vi "startup data collection.vi"(0 "Refnum in":T1, 1 "To Date":timestamp, 2 "Form Date":timestamp, 3 "Report filter":string, 5 "Shift":string, 7 "Select Line":string, 9 "columns":string[](array[string]), 11 "error in (no error)":errorcluster, 12 "Select Year":string, 13 "Select Month":string, 14 "table":string) -> (4 "Refnum out":T1, 6 "Array":string[](array[string]), 8 "Elements Found out":string[](array[string]), 10 "size(s)":i32, 15 "error out":errorcluster)   [LabVIEW 2017]
uses:
  <vilib>/addons/database/Connection.llb/Conn ObjectReference.ctl
  <vilib>/addons/database/NI_Database_API.lvlib
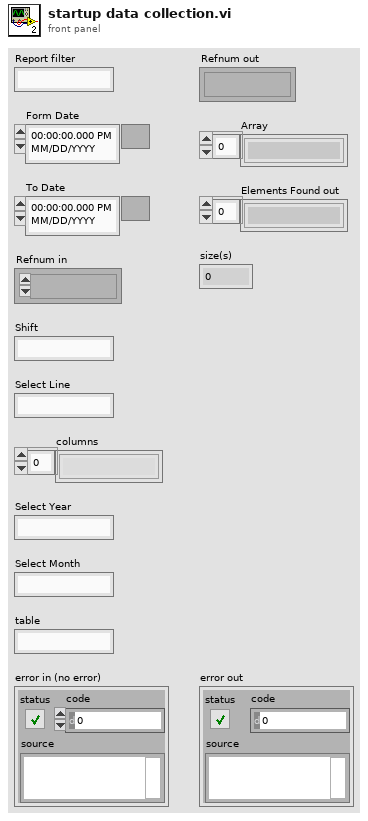
[diagram p1: front panel]
types:
  T1 = typedef "NI_Database_API.lvlib/Conn ObjectReference.ctl" = refnum<k1>
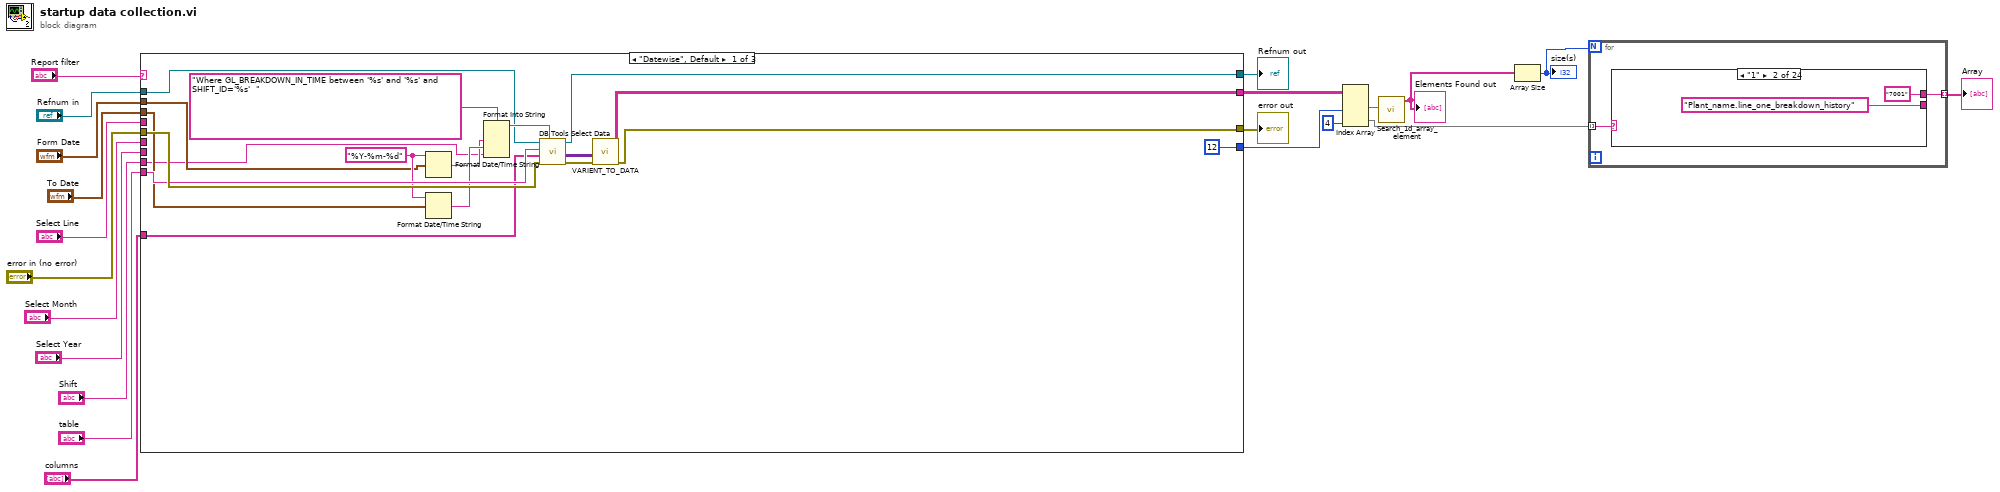
[diagram p0: block diagram]
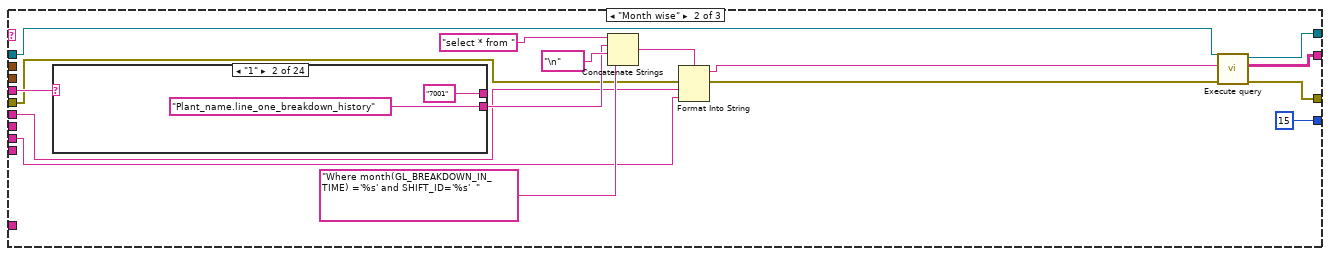
[diagram p2: hidden frame]
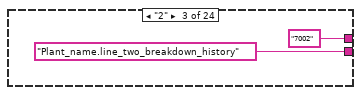
[diagram p4: hidden frame]
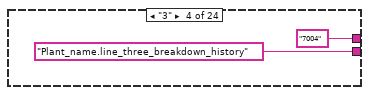
[diagram p5: hidden frame]
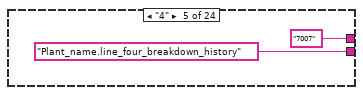
[diagram p6: hidden frame]
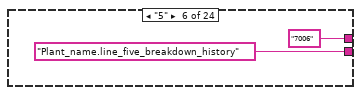
[diagram p7: hidden frame]
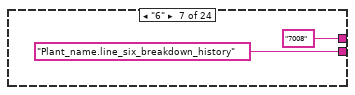
[diagram p8: hidden frame]
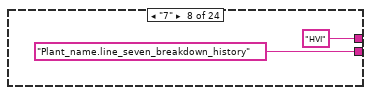
[diagram p9: hidden frame]
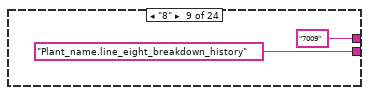
[diagram p10: hidden frame]
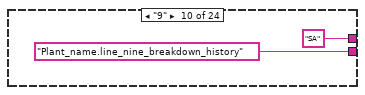
[diagram p11: hidden frame]
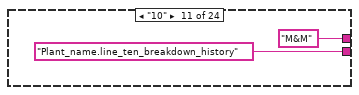
[diagram p12: hidden frame]
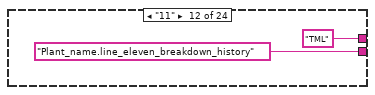
[diagram p13: hidden frame]
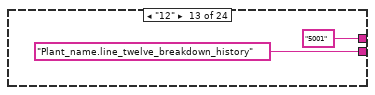
[diagram p14: hidden frame]
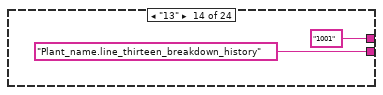
[diagram p15: hidden frame]
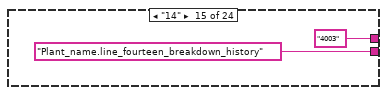
[diagram p16: hidden frame]
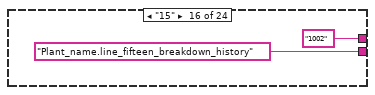
[diagram p17: hidden frame]
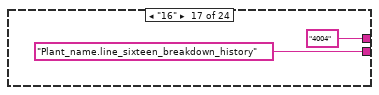
[diagram p18: hidden frame]
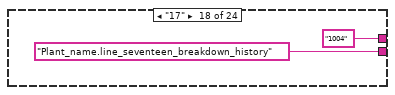
[diagram p19: hidden frame]
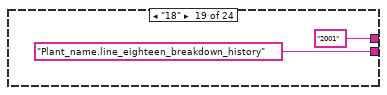
[diagram p20: hidden frame]
diagram:
  n1 = case shown="\"Datewise\", Default" "Report filter" {
    tunnel: [w37 w49 w102] -> w1
    tunnel: "Refnum in" -> [w36 w46 w113]
    tunnel: [w35 w48 w114] -> w9
    tunnel: "error in (no error)" -> [w34 w41 w109]
    tunnel: "table" -> [w33 _ _]
    tunnel: "columns" -> [w32 _ _]
    tunnel: [w30 w43 w112] -> w13
    tunnel: "Form Date" -> [w25 _ _]
    tunnel: "To Date" -> [w24 _ _]
    tunnel: "Shift" -> [w23 w45 w107]
    tunnel: "Select Line" -> [_ w51 w104]
    tunnel: "Select Month" -> [_ w44 _]
    tunnel: [12 ("disabled index (col)") 15 ("disabled index (col)") 15 ("disabled index (col)")] -> w20
    tunnel: "Select Year" -> [_ _ w108]
    frame "Datewise", Default {
      w29 = "%Y-%m-%d" ("time format string (%c)")
      n2 = Format Date/Time String(time format string (%c)=w29, seconds (now)=w25) -> (date/time string=w27:string)  [unwired: 1 in]
      n3 = Format Date/Time String(time format string (%c)=w29, seconds (now)=w24) -> (date/time string=w28:string)  [unwired: 1 in]
      n4 = Format Into String(format string="Where GL_BREAKDOWN_IN_TIME between '%s' and '%s' and SHIFT_ID='%s'  " ("condition"), w27, w28, w23) -> (resulting string=w39:string)  [unwired: 2 in, 1 out]
      n5 = call <vilib>:"DB Tools Select Data.vi"("condition"=w39, "error in (no error)"=w34, "columns"=w32, "table"=w33, "connection reference"=w36) -> ("error out"=w31:errorcluster, "data"=w38:variant[][], "connection reference out"=w35:T1)  [unwired: 1 in]
      n6 = call "VARIENT_TO_DATA.vi"("data"=w38, "error in (no error)"=w31) -> ("Table"=w37:string[][], "error out"=w30:errorcluster)  [unwired: 7 in]
    }
    frame "Month wise" {
      n7 = case shown="\"1\"" w51 {
        tunnel: [_ "7001" "7002" "7004" "7007" "7006" "7008" "HVI" "7009" "SA" "M&M" "TML" "5001" "1001" "4003" "1002" "4004" "1004" "2001" "3001" "2004" "3002" "3003" "4001"] -> _
        tunnel: [_ "Plant_name.line_one_breakdown_history" ("table") "Plant_name.line_two_breakdown_history" ("table") "Plant_name.line_three_breakdown_history" ("table") "Plant_name.line_four_breakdown_history" ("table") "Plant_name.line_five_breakdown_history" ("table") "Plant_name.line_six_breakdown_history" ("table") "Plant_name.line_seven_breakdown_history" ("table") "Plant_name.line_eight_breakdown_history" ("table") "Plant_name.line_nine_breakdown_history" ("table") "Plant_name.line_ten_breakdown_history" ("table") "Plant_name.line_eleven_breakdown_history" ("table") "Plant_name.line_twelve_breakdown_history" ("table") "Plant_name.line_thirteen_breakdown_history" ("table") "Plant_name.line_fourteen_breakdown_history" ("table") "Plant_name.line_fifteen_breakdown_history" ("table") "Plant_name.line_sixteen_breakdown_history" ("table") "Plant_name.line_seventeen_breakdown_history" ("table") "Plant_name.line_eighteen_breakdown_history" ("table") "Plant_name.line_nineteen_breakdown_history" ("table") "Plant_name.line_twenty_breakdown_history" ("table") "Plant_name.line_twenty_one_breakdown_history" ("table") "Plant_name.line_twenty_two_breakdown_history" ("table") "Plant_name.line_twenty_three_breakdown_history" ("table")] -> w50
        frame "0", Default {
        }
        frame "1" {
        }
        frame "2" {
        }
        frame "3" {
        }
        frame "4" {
        }
        frame "5" {
        }
        frame "6" {
        }
        frame "7" {
        }
        frame "8" {
        }
        frame "9" {
        }
        frame "10" {
        }
        frame "11" {
        }
        frame "12" {
        }
        frame "13" {
        }
        frame "14" {
        }
        frame "15" {
        }
        frame "16" {
        }
        frame "17" {
        }
        frame "18" {
        }
        frame "19" {
        }
        frame "20" {
        }
        frame "21" {
        }
        frame "22" {
        }
        frame "23" {
        }
      }
      n8 = Concatenate Strings("select * from " ("string"), w50, "\n" ("string"), "Where month(GL_BREAKDOWN_IN_TIME) ='%s' and SHIFT_ID='%s'  " ("condition")) -> (w52:string)
      n9 = Format Into String(format string=w52, error in=w41, w44, w45) -> (resulting string=w47:string, error out=w42:errorcluster)  [unwired: 1 in]
      n10 = call "Execute query.vi"("error in (no error)"=w42, "String"=w47, "connection reference"=w46) -> ("error out"=w43:errorcluster, "Table"=w49:string[][], "connection reference 2"=w48:T1)  [unwired: 5 in, 1 out]
    }
    frame "Year wise" {
      n11 = case shown="\"1\"" w104 {
        tunnel: [_ "7001" "7002" "7004" "7007" "7006" "7008" "HVI" "7009" "SA" "M&M" "TML" "5001" "1001" "4003" "1002" "4004" "1004" "2001" "3001" "2004" "3002" "3003" "4001"] -> _
        tunnel: [string[] ["Plant_name.line_one_breakdown_history", "Plant_name.line_two_breakdown_history", "Plant_name.line_three_breakdown_history", "Plant_name.line_four_breakdown_history", "Plant_name.line_five_breakdown_history", "Plant_name.line_six_breakdown_history", "Plant_name.line_seven_breakdown_history", "Plant_name.line_eight_breakdown_history", "Plant_name.line_nine_breakdown_history", "Plant_name.line_ten_breakdown_history", "Plant_name.line_eleven_breakdown_history", "Plant_name.line_eleven_breakdown_history", "Plant_name.line_twelve_breakdown_history", "Plant_name.line_thirteen_breakdown_history", "Plant_name.line_fourteen_breakdown_history", "Plant_name.line_fifteen_breakdown_history", "Plant_name.line_sixteen_breakdown_history", "Plant_name.line_seventeen_breakdown_history", "Plant_name.line_eighteen_breakdown_history", "Plant_name.line_nineteen_breakdown_history", "Plant_name.line_twenty_breakdown_history", "Plant_name.line_twenty_one_breakdown_history", "Plant_name.line_twenty_two_breakdown_history", "Plant_name.line_twenty_three_breakdown_history"] string[] ["      Plant_name.line_one_breakdown_history"] string[] ["Plant_name.line_two_breakdown_history"] string[] ["Plant_name.line_three_breakdown_history"] string[] ["Plant_name.line_four_breakdown_history"] string[] ["Plant_name.line_five_breakdown_history"] string[] ["Plant_name.line_six_breakdown_history"] string[] ["Plant_name.line_seven_breakdown_history"] string[] ["Plant_name.line_eight_breakdown_history"] string[] ["Plant_name.line_nine_breakdown_history"] string[] ["Plant_name.line_ten_breakdown_history"] string[] ["Plant_name.line_eleven_breakdown_history"] string[] ["Plant_name.line_twelve_breakdown_history"] string[] ["Plant_name.line_thirteen_breakdown_history"] string[] ["Plant_name.line_fourteen_breakdown_history"] string[] ["Plant_name.line_fifteen_breakdown_history"] string[] ["Plant_name.line_sixteen_breakdown_history"] string[] ["Plant_name.line_seventeen_breakdown_history"] string[] ["Plant_name.line_eighteen_breakdown_history"] string[] ["Plant_name.line_nineteen_breakdown_history"] string[] ["Plant_name.line_twenty_breakdown_history"] string[] ["Plant_name.line_twenty_one_breakdown_history"] string[] ["Plant_name.line_twenty_two_breakdown_history"] string[] ["Plant_name.line_twenty_three_breakdown_history"]] -> w110
        frame "ALL", Default {
        }
        frame "1" {
        }
        frame "2" {
        }
        frame "3" {
        }
        frame "4" {
        }
        frame "5" {
        }
        frame "6" {
        }
        frame "7" {
        }
        frame "8" {
        }
        frame "9" {
        }
        frame "10" {
        }
        frame "11" {
        }
        frame "12" {
        }
        frame "13" {
        }
        frame "14" {
        }
        frame "15" {
        }
        frame "16" {
        }
        frame "17" {
        }
        frame "18" {
        }
        frame "19" {
        }
        frame "20" {
        }
        frame "21" {
        }
        frame "22" {
        }
        frame "23" {
        }
      }
      n12 = case shown="\"ALL\"" w104 {
        tunnel: w110 -> [w121 w138]
        tunnel: w109 -> [w120 w137]
        tunnel: w108 -> [w119 w136]
        tunnel: w107 -> [w118 w135]
        tunnel: [w117 w134] -> w106
        tunnel: [w116 w133] -> w105
        frame "False", Default {
          n13 = for {
            tunnel: w121 -> [w128] mode=indexing
            tunnel: w119 -> [w125]
            tunnel: w118 -> [w124]
            tunnel: "Where year(GL_BREAKDOWN_IN_TIME) ='%s' and SHIFT_ID='%s'  " ("condition") -> [w130]
            tunnel: [w123] -> w117 mode=indexing
            tunnel: w120 -> [w126]
            tunnel: [w122] -> w116
            n14 = Concatenate Strings("select * from " ("string"), w128, "\n" ("string"), w130) -> (w127:string)
            n15 = Format Into String(format string=w127, error in=w126, w125, w124) -> (resulting string=w123:string, error out=w122:errorcluster)  [unwired: 1 in]
          }
        }
        frame "ALL" {
          n16 = for {
            tunnel: w138 -> [w145] mode=indexing
            tunnel: w136 -> [w142]
            tunnel: w135 -> [w141]
            tunnel: "Where year(GL_BREAKDOWN_IN_TIME) ='%s' and SHIFT_ID='%s'  " ("condition") -> [w147]
            tunnel: [w140] -> w134 mode=indexing
            tunnel: w137 -> [w143]
            tunnel: [w139] -> w133
            n17 = Concatenate Strings("select * from " ("string"), w145, "\n" ("string"), w147) -> (w144:string)
            n18 = Format Into String(format string=w144, error in=w143, w142, w141) -> (resulting string=w140:string, error out=w139:errorcluster)  [unwired: 1 in]
          }
        }
      }
      n19 = for {
        tunnel: [w196] -> _
        tunnel: w113 -> [w202]
        tunnel: [w203] -> w114
        tunnel: [w201] -> w112
        tunnel: w106 -> [w200] mode=indexing
        tunnel: w105 -> [w199]
        shift-right: [w198] -> w102
        shift-left: string[][] [] -> [w197]
        n20 = call "Execute query.vi"("error in (no error)"=w199, "String"=w200, "connection reference"=w202) -> ("error out"=w201:errorcluster, "Table"=w196:string[][], "connection reference 2"=w203:T1)  [unwired: 5 in, 1 out]
        n21 = Build Array (concatenate)(w197, w196) -> (w198:string[][])
      }
    }
  }
  "error out" <- w13
  "Refnum out" <- w9
  n22 = Index Array(array=w1, index (col) #1=w20, index (col) #2=4 ("index (col)")) -> (element #1=w3:string[], element #2=w4:string[])  [unwired: 2 in]
  n23 = call "Search_1d_array_element.vi"("BD Date"=w3) -> ("Elements Found out"=w6:string[])  [unwired: 6 in, 2 out]
  "Elements Found out" <- w6
  n24 = Array Size(array=w6) -> (size(s)=w5:i32)
  "size(s)" <- w5
  n25 = for {
    N: w5 -> [_]
    tunnel: w4 -> [w205] mode=indexing
    tunnel: [w204] -> w7 mode=indexing
    n26 = case shown="\"1\"" w205 {
      tunnel: ["" "7001" "7002" "7004" "7007" "7006" "7008" "HVI" "7009" "SA" "M&M" "TML" "5001" "1001" "4003" "1002" "4004" "1004" "2001" "3001" "2004" "3002" "3003" "4001"] -> w204
      tunnel: [_ "Plant_name.line_one_breakdown_history" ("table") "Plant_name.line_two_breakdown_history" ("table") "Plant_name.line_three_breakdown_history" ("table") "Plant_name.line_four_breakdown_history" ("table") "Plant_name.line_five_breakdown_history" ("table") "Plant_name.line_six_breakdown_history" ("table") "Plant_name.line_seven_breakdown_history" ("table") "Plant_name.line_eight_breakdown_history" ("table") "Plant_name.line_nine_breakdown_history" ("table") "Plant_name.line_ten_breakdown_history" ("table") "Plant_name.line_eleven_breakdown_history" ("table") "Plant_name.line_twelve_breakdown_history" ("table") "Plant_name.line_thirteen_breakdown_history" ("table") "Plant_name.line_fourteen_breakdown_history" ("table") "Plant_name.line_fifteen_breakdown_history" ("table") "Plant_name.line_sixteen_breakdown_history" ("table") "Plant_name.line_seventeen_breakdown_history" ("table") "Plant_name.line_eighteen_breakdown_history" ("table") "Plant_name.line_nineteen_breakdown_history" ("table") "Plant_name.line_twenty_breakdown_history" ("table") "Plant_name.line_twenty_one_breakdown_history" ("table") "Plant_name.line_twenty_two_breakdown_history" ("table") "Plant_name.line_twenty_three_breakdown_history" ("table")] -> _
      frame "0", Default {
      }
      frame "1" {
      }
      frame "2" {
      }
      frame "3" {
      }
      frame "4" {
      }
      frame "5" {
      }
      frame "6" {
      }
      frame "7" {
      }
      frame "8" {
      }
      frame "9" {
      }
      frame "10" {
      }
      frame "11" {
      }
      frame "12" {
      }
      frame "13" {
      }
      frame "14" {
      }
      frame "15" {
      }
      frame "16" {
      }
      frame "17" {
      }
      frame "18" {
      }
      frame "19" {
      }
      frame "20" {
      }
      frame "21" {
      }
      frame "22" {
      }
      frame "23" {
      }
    }
  }
  "Array" <- w7
